vi "Config Timer.vi"(0 "VISA resource name":refnum<visa-resource-name>, 1 "Count (1)":u32=1, 2 "Delay (1e-3)":dbl=0.001, 3 "Delay List":dbl[](array[numeric]) min=0.0, 5 "Node In":string, 7 "Timer Number (1)":u32=1 min=1 max=10, 9 "Passthrough (Off)":bool, 11 "error in":errorcluster, 12 "Input Event":string="0") -> (4 "VISA resource name out":refnum<visa-resource-name>, 6 "Node Out":string, 14 "Command String":string, 15 "error out":errorcluster)   [LabVIEW 2009, in "Keithley 2600 Series.lvlib"]
doc: "This VI configures a timer in the advanced trigger model.\n\n<b>Remarks:</b>\nThe reception of an event by a timer will cause a delay to be initiated. Upon the expiration of this timer an output event will be generated.\n\n<b>Functions and Attributes Used</b>\ntrigger.timer[n].count\ntrigger.timer[n].delay\ntrigger.timer[n].delaylist\ntrigger.timer[n].passthrough\ntrigger.timer[n].stimulus"
uses:
  <instrlib>/Keithley 2600 Series/Keithley 2600 Series.lvlib
  <instrlib>/Keithley 2600 Series/Private/GlobalVariables.vi
panel:
  # "(c) 2008 Keithley Instruments, Inc.  ALL RIGHTS RESERVED."
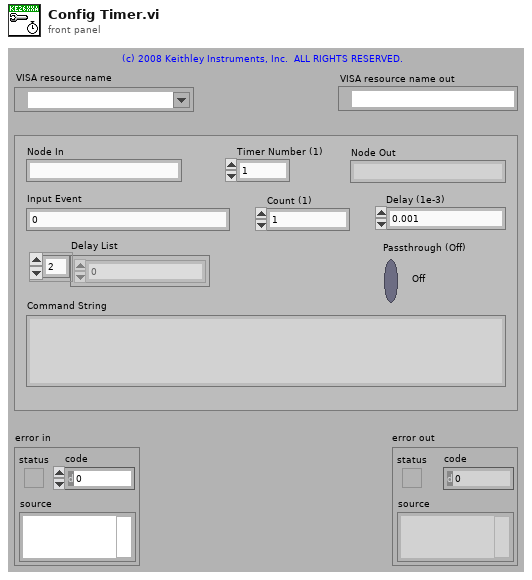
[diagram p1: front panel]
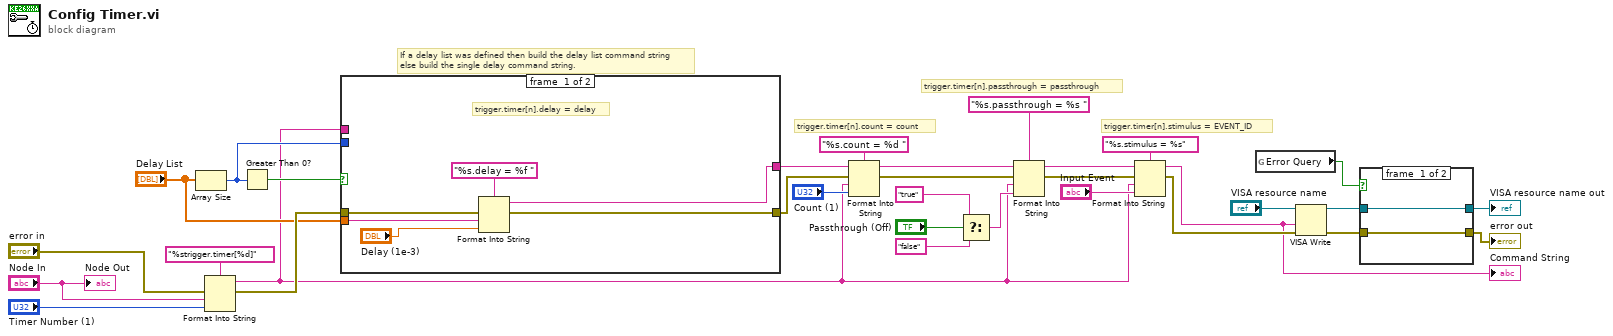
[diagram p0: block diagram]
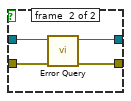
[diagram p2: hidden frame]
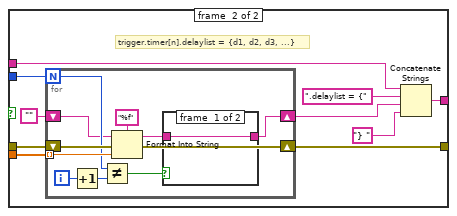
[diagram p3: hidden frame]
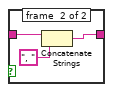
[diagram p4: hidden frame]
diagram:
  # "trigger.timer[n].stimulus = EVENT_ID"
  # "trigger.timer[n].passthrough = passthrough"
  # "trigger.timer[n].count = count"
  # "If a delay list was defined then build the delay list command string\nelse build the single delay command string."
  n1 = Array Size(array="Delay List") -> (size(s)=w25:i32)
  n2 = Format Into String(format string="%strigger.timer[%d]", error in="error in", "Node In", "Timer Number (1)") -> (resulting string=w9:string, error out=w27:errorcluster)  [unwired: 1 in]
  n3 = Greater Than 0?(x=w25) -> (x > 0?=w32:bool)
  n4 = case shown="True" w32 {
    tunnel: w9 -> [w36 w41]
    tunnel: w27 -> [w35 w45]
    tunnel: [w34 w44] -> w17
    tunnel: [w33 w40] -> w21
    tunnel: "Delay List" -> [_ w46]
    tunnel: w25 -> [_ w47]
    frame #0 {
      # "trigger.timer[n].delay = delay"
      n5 = Format Into String(format string="%s.delay = %f ", error in=w35, w36, "Delay (1e-3)") -> (resulting string=w33:string, error out=w34:errorcluster)  [unwired: 1 in]
    }
    frame #1 {
      # "trigger.timer[n].delaylist = {d1, d2, d3, ...}"
      n6 = for {
        N: w47 -> [w55]
        tunnel: w46 -> [w58] mode=indexing
        shift-right: [w52] -> w44
        shift-left: w45 -> [w57]
        shift-right: [w53] -> w42
        shift-left: "" -> [w49]
        i -> [w51]
        n7 = Increment(x=w51) -> (x+1=w50:i32)
        n8 = Not Equal?(x=w55, y=w50) -> (x != y?=w54:bool)
        n9 = Format Into String(format string="%f", initial string=w49, error in=w57, w58) -> (resulting string=w56:string, error out=w52:errorcluster)
        n10 = case shown="True" w54 {
          tunnel: w56 -> [w60 w62]
          tunnel: [w60 w61] -> w53
          frame #0 {
          }
          frame #1 {
            n11 = Concatenate Strings(w62, ", " ("string")) -> (w61:string)
          }
        }
      }
      n12 = Concatenate Strings(w41, ".delaylist = {" ("format string"), w42, "} " ("string")) -> (w40:string)
    }
  }
  n13 = Format Into String(format string="%s.count = %d ", initial string=w21, error in=w17, w9, "Count (1)") -> (resulting string=w20:string, error out=w12:errorcluster)
  n14 = Select(t="true", s="Passthrough (Off)", f="false") -> (s? t:f=w13:string)
  n15 = Format Into String(format string="%s.passthrough = %s ", initial string=w20, error in=w12, w9, w13) -> (resulting string=w19:string, error out=w11:errorcluster)
  n16 = Format Into String(format string="%s.stimulus = %s", initial string=w19, error in=w11, w9, "Input Event") -> (resulting string=w1:string, error out=w8:errorcluster)
  "Command String" <- w1
  n17 = global read "GlobalVariables.vi" "Error Query"() -> (w6:bool)
  n18 = VISA Write(VISA resource name="VISA resource name", write buffer=w1, error in (no error)=w8) -> (VISA resource name out=w5:refnum<visa-resource-name>, error out=w4:errorcluster)  [unwired: 1 out]
  n19 = case shown="True" w6 {
    tunnel: w5 -> [w65 w69]
    tunnel: w4 -> [w64 w68]
    tunnel: [w65 w67] -> w3
    tunnel: [w64 w66] -> w2
    frame #0 {
    }
    frame #1 {
      n20 = call <instrlib>:"Error Query.vi"("error in (no error)"=w68, "VISA resource name"=w69) -> ("error out"=w66:errorcluster, "VISA resource name out"=w67:refnum<visa-resource-name>)  [unwired: 8 out]
    }
  }
  "VISA resource name out" <- w3
  "error out" <- w2
  "Node Out" <- "Node In"
